vi "Initialize.vi"() -> (14 "State Out":T1 {"BlockNodeState"."Draw Style" items=["FunctionBlock", "ExpressVI", "Variable", "Elemental I/O", "32x32 Icon", "FunctionBlockCompact"]; "BlockNodeState"."Terminal Data"."Terminal Flags" format="%.0b"})   [LabVIEW 2020, in "NI_ExpressFull.lvlib" / "ExpressSpectralMeasurementsBlockNode.xnode"]
uses:
  <vilib>/express/express analysis/Spectral/XNode/ExpressSpectralMeasurementsBlockNode.xnode
  <vilib>/express/express analysis/Spectral/XNode/State.ctl
  <vilib>/BlockNodeSupport/BlockNodeState.ctl
  <vilib>/picture/picture.llb/imagedata.ctl
  <vilib>/express/express shared/XNodes/controls/ExpressState.ctl
  <vilib>/BlockNodeSupport/TerminalData.ctl
  <vilib>/XNodeSupport/XNodeType.ctl
  <vilib>/XNodeSupport/NI_XNodeSupport.lvlib
  <vilib>/express/express shared/XNodes/controls/ExpressTerminalInfo.ctl
panel:
  in  "config path":path=path "<vilib>/express/express analysis/Spectral/Config/ExnSpectralConfig Configure Spectral Measurements.vi"
  in  "block VI path":path=path "<vilib>/express/express analysis/Spectral/Block/ExnSpectralBlock spectral measurements.vi"
  in  "State In":T1={"BlockNodeState"={"Terminal Data"=[{"Terminal Name"="Signals", "Terminal Display Name"="Signals", "Terminal ID"="Signals", "Terminal Flags"=517, "Terminal Type"=variant(waveform(dbl) {"t0"=timestamp(0 s since 1904-01-01), "dt"=0.0, "Y"=[]}), "Terminal Map ID"=0}, {"Terminal Name"="Selected Measurements", "Terminal Display Name"="Selected Measurements", "Terminal ID"="Selected Measurements", "Terminal Flags"=769, "Terminal Type"=variant(u32 0), "Terminal Map ID"=1}, {"Terminal Name"="Restart Averaging", "Terminal Display Name"="Restart Averaging", "Terminal ID"="Restart Averaging", "Terminal Flags"=769, "Terminal Type"=variant(bool FALSE), "Terminal Map ID"=2}, {"Terminal Name"="View", "Terminal Display Name"="View", "Terminal ID"="View", "Terminal Flags"=769, "Terminal Type"=variant(cluster{"dB On (F)":bool, "unwrap phase (F)":bool, "convert to degree (F)":bool} {"dB On (F)"=TRUE, "unwrap phase (F)"=FALSE, "convert to degree (F)"=FALSE}), "Terminal Map ID"=3}, {"Terminal Name"="Spectrum Window", "Terminal Display Name"="Spectrum Window", "Terminal ID"="Spectrum Window", "Terminal Flags"=769, "Terminal Type"=variant(u16 1), "Terminal Map ID"=4}, {"Terminal Name"="Spectrum Averaging Parameters", "Terminal Display Name"="Spectrum Averaging Parameters", "Terminal ID"="Spectrum Averaging Parameters", "Terminal Flags"=769, "Terminal Type"=variant(cluster{"averaging mode":u16, "weighting mode":u16, "number of averages":u32} {"averaging mode"=0, "weighting mode"=1, "number of averages"=10}), "Terminal Map ID"=5}, {"Terminal Name"="All Spectra", "Terminal Display Name"="All Spectra", "Terminal ID"="All Spectra", "Terminal Flags"=769, "Terminal Type"=variant(bool TRUE), "Terminal Map ID"=6}, {"Terminal Name"="error in (no error)", "Terminal Display Name"="error in (no error)", "Terminal ID"="error in (no error)", "Terminal Flags"=513, "Terminal Type"=variant(errorcluster {"status"=FALSE, "code"=0, "source"=""}), "Terminal Map ID"=7}, {"Terminal Name"="Measurement Output", "Terminal Display Name"="Measurement Output", "Terminal ID"="Measurement Output", "Terminal Flags"=525, "Terminal Type"=variant(dynamicdata []), "Terminal Map ID"=8}, {"Terminal Name"="averaging done", "Terminal Display Name"="averaging done", "Terminal ID"="averaging done", "Terminal Flags"=777, "Terminal Type"=variant(bool FALSE), "Terminal Map ID"=9}, {"Terminal Name"="Phase", "Terminal Display Name"="Phase", "Terminal ID"="Phase", "Terminal Flags"=525, "Terminal Type"=variant(dynamicdata []), "Terminal Map ID"=10}, {"Terminal Name"="error out", "Terminal Display Name"="error out", "Terminal ID"="error out", "Terminal Flags"=521, "Terminal Type"=variant(errorcluster {"status"=FALSE, "code"=0, "source"=""}), "Terminal Map ID"=11}], "Instance Name"="Spectral Measurements", "Type Name"="Spectral Measurements", "Draw Style"=1, "Connector Pane Pattern"=4833, "Flags"=370, "Grown Terminal List Order"=[], "Image"={"image type"=0, "image depth"=8, "image"=[0, 0, 255, 255, 255, 255, 255, 255, 255, 255, 255, 255, 255, 255, 255, 255, 255, 255, 255, 255, 255, 255, 255, 255, 255, 255, 255, 255, 255, 255, 0, 0, 0, 255, 210, 210, 210, 210, 210, 210, 210, 210, 210, 210, 210, 210, 210, 210, 210, 210, 210, 210, 210, 210, 210, 210, 210, 210, 210, 210, 210, 210, 255, 0, 255, 210, 210, 210, 210, 210, 210, 210, 210, 210, 210, 210, 210, 210, 210, 210, 210, 210, 210, 210, 210, 210, 210, 210, 210, 210, 210, 210, 210, 210, 210, 255, 255, 0, 0, 0, 0, 0, 0, 0, 0, 0, 0, 0, 0, 0, 0, 0, 0, 0, 0, 0, 0, 0, 0, 0, 0, 0, 0, 0, 0, 0, 0, 255, 255, 0, 0, 0, 0, 0, 0, 0, 0, 0, 0, 0, 0, 0, 0, 0, 0, 0, 0, 0, 0, 0, 0, 0, 0, 0, 0, 0, 0, 0, 0, 255, 255, 0, 0, 0, 0, 0, 0, 0, 0, 0, 0, 0, 0, 0, 0, 86, 86, 86, 86, 86, 86, 86, 86, 86, 86, 86, 86, 86, 86, 86, 86, 255, 255, 0, 0, 0, 0, 0, 0, 0, 0, 0, 0, 0, 0, 0, 0, 255, 255, 255, 255, 255, 255, 255, 255, 255, 255, 255, 255, 255, 255, 255, 255, 255, 255, 0, 0, 250, 250, 0, 0, 0, 0, 0, 0, 0, 0, 0, 0, 255, 5, 5, 5, 5, 5, 5, 5, 5, 5, 5, 5, 5, 5, 5, 5, 255, 255, 0, 0, 0, 250, 0, 0, 0, 0, 0, 0, 0, 0, 0, 0, 255, 5, 255, 5, 5, 5, 255, 5, 5, 5, 255, 5, 5, 5, 255, 5, 255, 255, 0, 0, 0, 250, 0, 0, 0, 0, 0, 0, 0, 0, 0, 0, 255, 5, 255, 5, 255, 5, 255, 5, 255, 5, 255, 5, 255, 5, 255, 5, 255, 255, 0, 0, 0, 250, 0, 0, 0, 0, 0, 0, 0, 0, 0, 0, 255, 255, 255, 255, 255, 255, 255, 255, 255, 255, 255, 255, 255, 255, 255, 255, 255, 255, 0, 0, 250, 250, 0, 0, 0, 0, 0, 0, 0, 0, 0, 0, 0, 0, 0, 0, 0, 0, 0, 0, 0, 0, 0, 0, 0, 0, 0, 0, 255, 255, 0, 0, 0, 250, 0, 0, 0, 0, 0, 0, 0, 0, 0, 0, 0, 0, 0, 0, 0, 0, 0, 0, 0, 0, 0, 0, 0, 0, 0, 0, 255, 255, 0, 0, 0, 250, 0, 0, 0, 0, 0, 0, 0, 0, 0, 0, 0, 0, 0, 0, 0, 0, 0, 0, 0, 0, 0, 0, 0, 0, 0, 0, 255, 255, 0, 0, 0, 250, 0, 0, 0, 0, 255, 0, 0, 0, 0, 0, 0, 0, 0, 0, 0, 0, 0, 0, 0, 0, 0, 0, 0, 0, 0, 0, 255, 255, 0, 0, 250, 250, 0, 0, 0, 0, 255, 0, 0, 0, 0, 0, 0, 0, 0, 0, 0, 0, 0, 0, 0, 0, 0, 0, 0, 0, 0, 0, 255, 255, 0, 0, 0, 250, 0, 0, 0, 0, 255, 0, 0, 0, 0, 0, 0, 0, 0, 0, 0, 0, 0, 0, 0, 0, 0, 0, 0, 0, 0, 0, 255, 255, 0, 0, 0, 250, 0, 0, 0, 0, 255, 0, 0, 0, 0, 0, 0, 0, 0, 0, 0, 0, 0, 0, 0, 0, 0, 0, 0, 0, 0, 0, 255, 255, 0, 0, 0, 250, 0, 0, 0, 0, 255, 0, 0, 0, 0, 0, 0, 0, 0, 0, 0, 0, 0, 0, 0, 0, 0, 0, 0, 0, 0, 0, 255, 255, 0, 0, 250, 250, 0, 0, 0, 0, 255, 0, 0, 0, 0, 0, 0, 0, 0, 0, 0, 0, 0, 0, 0, 0, 0, 0, 0, 0, 0, 0, 255, 255, 0, 0, 0, 250, 0, 0, 0, 255, 255, 255, 0, 0, 0, 0, 0, 0, 0, 0, 0, 0, 0, 0, 0, 0, 0, 0, 0, 0, 0, 0, 255, 255, 0, 0, 0, 250, 0, 0, 0, 255, 255, 255, 0, 0, 0, 0, 0, 0, 0, 0, 0, 0, 0, 0, 0, 0, 0, 0, 0, 0, 0, 0, 255, 255, 0, 0, 0, 250, 0, 0, 0, 255, 255, 255, 255, 0, 0, 0, 0, 0, 0, 0, 0, 0, 0, 0, 0, 0, 0, 0, 0, 0, 0, 0, 255, 255, 0, 0, 250, 250, 0, 0, 255, 255, 0, 0, 255, 0, 0, 0, 0, 0, 0, 0, 0, 0, 0, 0, 0, 0, 0, 0, 0, 0, 0, 0, 255, 255, 0, 0, 0, 250, 255, 255, 255, 255, 0, 0, 255, 255, 0, 0, 0, 0, 0, 0, 0, 0, 0, 0, 0, 0, 0, 0, 0, 0, 0, 0, 255, 255, 0, 0, 0, 250, 0, 255, 0, 0, 0, 0, 0, 255, 255, 255, 255, 255, 255, 255, 255, 255, 255, 255, 255, 255, 255, 255, 0, 0, 0, 0, 255, 255, 0, 0, 0, 250, 0, 0, 0, 0, 0, 0, 0, 0, 0, 0, 0, 0, 0, 0, 0, 0, 0, 0, 0, 0, 0, 0, 0, 0, 0, 0, 255, 255, 0, 0, 250, 250, 250, 250, 250, 250, 250, 250, 250, 250, 250, 250, 250, 250, 250, 250, 250, 250, 250, 250, 250, 250, 250, 250, 250, 250, 0, 0, 255, 255, 0, 0, 0, 250, 0, 0, 0, 250, 0, 0, 0, 250, 0, 0, 0, 250, 0, 0, 0, 250, 0, 0, 0, 250, 0, 0, 0, 250, 0, 0, 255, 255, 0, 0, 0, 0, 0, 0, 0, 0, 0, 0, 0, 0, 0, 0, 0, 0, 0, 0, 0, 0, 0, 0, 0, 0, 0, 0, 0, 0, 0, 0, 255, 0, 255, 0, 0, 0, 0, 0, 0, 0, 0, 0, 0, 0, 0, 0, 0, 0, 0, 0, 0, 0, 0, 0, 0, 0, 0, 0, 0, 0, 0, 255, 0, 0, 0, 255, 255, 255, 255, 255, 255, 255, 255, 255, 255, 255, 255, 255, 255, 255, 255, 255, 255, 255, 255, 255, 255, 255, 255, 255, 255, 255, 255, 0, 0], "mask"=[63, 255, 255, 252, 127, 255, 255, 254, 255, 255, 255, 255, 255, 255, 255, 255, 255, 255, 255, 255, 255, 255, 255, 255, 255, 255, 255, 255, 255, 255, 255, 255, 255, 255, 255, 255, 255, 255, 255, 255, 255, 255, 255, 255, 255, 255, 255, 255, 255, 255, 255, 255, 255, 255, 255, 255, 255, 255, 255, 255, 255, 255, 255, 255, 255, 255, 255, 255, 255, 255, 255, 255, 255, 255, 255, 255, 255, 255, 255, 255, 255, 255, 255, 255, 255, 255, 255, 255, 255, 255, 255, 255, 255, 255, 255, 255, 255, 255, 255, 255, 255, 255, 255, 255, 255, 255, 255, 255, 255, 255, 255, 255, 255, 255, 255, 255, 255, 255, 255, 255, 127, 255, 255, 254, 63, 255, 255, 252], "colors"=[16777215, 16777164, 16777113, 16777062, 16777011, 16776960, 16764159, 16764108, 16764057, 16764006, 16763955, 16763904, 16751103, 16751052, 16751001, 16750950, 16750899, 16750848, 16738047, 16737996, 16737945, 16737894, 16737843, 16737792, 16724991, 16724940, 16724889, 16724838, 16724787, 16724736, 16711935, 16711884, 16711833, 16711782, 16711731, 16711680, 13434879, 13434828, 13434777, 13434726, 13434675, 13434624, 13421823, 13421772, 13421721, 13421670, 13421619, 13421568, 13408767, 13408716, 13408665, 13408614, 13408563, 13408512, 13395711, 13395660, 13395609, 13395558, 13395507, 13395456, 13382655, 13382604, 13382553, 13382502, 13382451, 13382400, 13369599, 13369548, 13369497, 13369446, 13369395, 13369344, 10092543, 10092492, 10092441, 10092390, 10092339, 10092288, 10079487, 10079436, 10079385, 10079334, 10079283, 10079232, 10066431, 10066380, 10066329, 10066278, 10066227, 10066176, 10053375, 10053324, 10053273, 10053222, 10053171, 10053120, 10040319, 10040268, 10040217, 10040166, 10040115, 10040064, 10027263, 10027212, 10027161, 10027110, 10027059, 10027008, 6750207, 6750156, 6750105, 6750054, 6750003, 6749952, 6737151, 6737100, 6737049, 6736998, 6736947, 6736896, 6724095, 6724044, 6723993, 6723942, 6723891, 6723840, 6711039, 6710988, 6710937, 6710886, 6710835, 6710784, 6697983, 6697932, 6697881, 6697830, 6697779, 6697728, 6684927, 6684876, 6684825, 6684774, 6684723, 6684672, 3407871, 3407820, 3407769, 3407718, 3407667, 3407616, 3394815, 3394764, 3394713, 3394662, 3394611, 3394560, 3381759, 3381708, 3381657, 3381606, 3381555, 3381504, 3368703, 3368652, 3368601, 3368550, 3368499, 3368448, 3355647, 3355596, 3355545, 3355494, 3355443, 3355392, 3342591, 3342540, 3342489, 3342438, 3342387, 3342336, 65535, 65484, 65433, 65382, 65331, 65280, 52479, 52428, 52377, 52326, 52275, 52224, 39423, 39372, 39321, 39270, 39219, 39168, 26367, 26316, 26265, 26214, 26163, 26112, 13311, 13260, 13209, 13158, 13107, 13056, 255, 204, 153, 102, 51, 15597568, 14483456, 12255232, 11141120, 8912896, 7798784, 5570560, 4456448, 2228224, 1114112, 60928, 56576, 47872, 43520, 34816, 30464, 21760, 17408, 8704, 4352, 238, 221, 187, 170, 136, 119, 85, 68, 34, 17, 15658734, 14540253, 12303291, 11184810, 8947848, 7829367, 5592405, 4473924, 2236962, 1118481, 0], "Rectangle"={"left"=0, "top"=0, "right"=32, "bottom"=32}}}, "ExpressState"={"Terminal Info"=[{"types to adapt"=["ExpressData", "Waveform", "1D Array Waveform"], "show config value"=FALSE, "default type"=variant(waveform(dbl) {"t0"=timestamp(0 s since 1904-01-01), "dt"=0.0, "Y"=[]}), "display name control"=""}, {"types to adapt"=["Numeric"], "show config value"=FALSE, "default type"=variant(u32 0), "display name control"=""}, {"types to adapt"=["Boolean"], "show config value"=FALSE, "default type"=variant(bool FALSE), "display name control"=""}, {"types to adapt"=[""], "show config value"=FALSE, "default type"=variant(cluster{"dB On (F)":bool, "unwrap phase (F)":bool, "convert to degree (F)":bool} {"dB On (F)"=TRUE, "unwrap phase (F)"=FALSE, "convert to degree (F)"=FALSE}), "display name control"=""}, {"types to adapt"=["Numeric"], "show config value"=FALSE, "default type"=variant(u16 1), "display name control"=""}, {"types to adapt"=[""], "show config value"=FALSE, "default type"=variant(cluster{"averaging mode":u16, "weighting mode":u16, "number of averages":u32} {"averaging mode"=0, "weighting mode"=1, "number of averages"=10}), "display name control"=""}, {"types to adapt"=["Boolean"], "show config value"=FALSE, "default type"=variant(bool TRUE), "display name control"=""}, {"types to adapt"=[""], "show config value"=FALSE, "default type"=variant(errorcluster {"status"=FALSE, "code"=0, "source"=""}), "display name control"=""}, {"types to adapt"=["ExpressData"], "show config value"=FALSE, "default type"=variant(dynamicdata []), "display name control"="output name"}, {"types to adapt"=["Boolean"], "show config value"=FALSE, "default type"=variant(bool FALSE), "display name control"=""}, {"types to adapt"=["ExpressData"], "show config value"=FALSE, "default type"=variant(dynamicdata []), "display name control"=""}, {"types to adapt"=[""], "show config value"=FALSE, "default type"=variant(errorcluster {"status"=FALSE, "code"=0, "source"=""}), "display name control"=""}], "config control names"=[], "config data strings"=[], "config control data"=[], "units"=[], "configured?"=FALSE, "config VI path"=path "<vilib>/express/express analysis/Spectral/Config/ExnSpectralConfig Configure Spectral Measurements.vi", "block VI path"=path "<vilib>/express/express analysis/Spectral/Block/ExnSpectralBlock Spectral Measurements.vi", "config control labels"=[], "show config value menu"=FALSE, "config value menu setting"=FALSE, "context help labels"=["Selected Measurement"], "valid help labels"=[]}} {"BlockNodeState"."Draw Style" items=["FunctionBlock", "ExpressVI", "Variable", "Elemental I/O", "32x32 Icon", "FunctionBlockCompact"]; "BlockNodeState"."Terminal Data"."Terminal Flags" format="%.0b"}
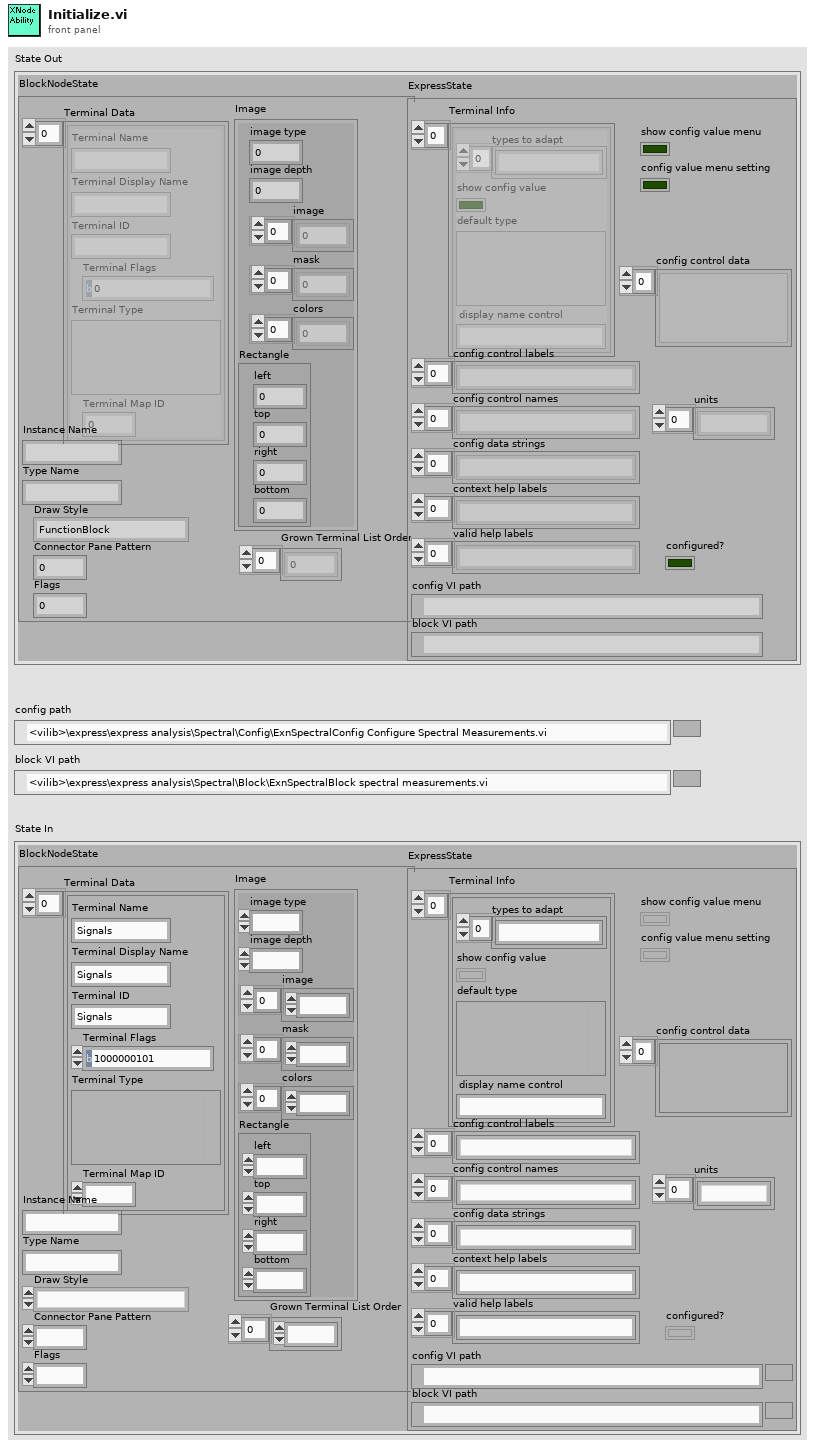
[diagram p1: front panel]
types:
  T1 = typedef "NI_ExpressFull.lvlib/ExpressSpectralMeasurementsBlockNode.xnode/State.ctl" = cluster{"BlockNodeState":T2, "ExpressState":T5}
  T2 = typedef "BlockNodeState.ctl" = cluster{"Terminal Data":T3[], "Instance Name":string, "Type Name":string, "Draw Style":i32, "Connector Pane Pattern":i32, "Flags":i32, "Grown Terminal List Order":i32[], "Image":T4}
  T3 = typedef "TerminalData.ctl" = cluster{"Terminal Name":string, "Terminal Display Name":string, "Terminal ID":string, "Terminal Flags":i32, "Terminal Type":variant, "Terminal Map ID":i32}
  T4 = typedef "imagedata.ctl" = cluster{"image type":i32, "image depth":i32, "image":u8[], "mask":u8[], "colors":u32[], "Rectangle":cluster{"left":i16, "top":i16, "right":i16, "bottom":i16}}
  T5 = typedef "ExpressState.ctl" = cluster{"Terminal Info":T6, "config control names":string[], "config data strings":string[], "config control data":variant[], "units":string[], "configured?":bool, "config VI path":path, "block VI path":path, "config control labels":string[], "show config value menu":bool, "config value menu setting":bool, "context help labels":string[], "valid help labels":string[]}
  T6 = typedef "ExpressTerminalInfo.ctl" = cluster{"types to adapt":string[], "show config value":bool, "default type":T7, "display name control":string}[]
  T7 = typedef "NI_XNodeSupport.lvlib/XNodeType.ctl" = variant
  T8 = typedef "ExpressBlockNodeState.ctl" = cluster{"BlockNodeState":T2, "ExpressState":T5}
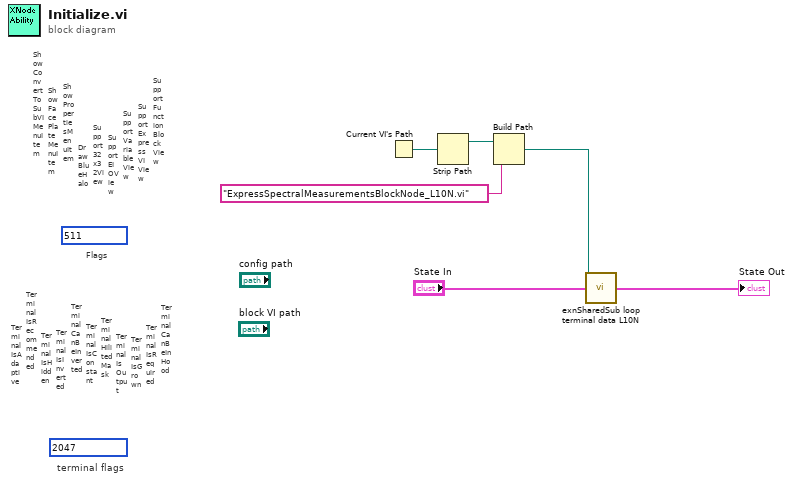
[diagram p0: block diagram]
diagram:
  (unwired) 511 ("BlockNodeState.nodeFlags")
  (unwired) 2047 ("TermFlags")
  # "ShowConvertToSubVIMenuItem"
  # "ShowFacePlateMenuItem"
  # "ShowPropertiesMenuItem"
  # "Flags"
  # "DrawBlueHalo"
  # "Support32x32View"
  # "SupportEIOView"
  # "SupportVariableView"
  # "SupportExpressVIView"
  # "SupportFunctionBlockView"
  # "TerminalIsAdaptive"
  # "TerminalIsRecommended"
  # "TerminalIsHidden"
  # "terminal flags"
  # "TerminalIsInverted"
  # "TerminalCanBeInverted"
  # "TerminalIsConstant"
  # "TerminalHilitedMask"
  # "TerminalIsOutput"
  # "TerminalIsGrown"
  # "TerminalIsRequired"
  # "TerminalCanBeInHood"
  n1 = Current VI's Path() -> (path=w5:path)
  n2 = Strip Path(path=w5) -> (stripped path=w4:path)  [unwired: 1 out]
  n3 = Build Path(base path=w4, name or relative path="ExpressSpectralMeasurementsBlockNode_L10N.vi") -> (appended path=w6:path)
  n4 = call <vilib>:"exnSharedSub loop terminal data L10N.vi"("path to L10N subVI"=w6, "ExpressBlockNodeState In"="State In") -> ("ExpressBlockNodeState Out"=→"State Out":T8)  [unwired: 13 out]
